vi "Humidifier CMD.vi"(8 "error in":errorcluster, 11 "cPAS in":refnum<class "cPAS.lvclass">) -> (0 "error out":errorcluster, 3 "cPAS out":refnum<class "cPAS.lvclass">)   [LabVIEW 2015, in "cPAS.lvclass"]
doc: "This VI responds to changes in the TEC Setpoint and the TEC enable for the PAS saturator. If the switch <B>RHctl</B> is set and the TEC is enabled, then the system will control the temperature setpoint based on a RH setpoint."
uses:
  cPAS.lvclass
  cPAS.lvclass/cPAS.ctl
  <vilib>/DAQmx/write.llb/DAQmx Write (Digital 1D Bool NChan 1Samp 1Line).vi
  <vilib>/DAQmx/write.llb/DAQmx Write (Analog 1D DBL NChan 1Samp).vi
  <vilib>/DAQmx/miscellaneous.llb/DAQmx Fill In Error Info.vi
  Reusable/PAS/Main/Read Data.vi
  Reusable/PAS/Data/Main/Write Current Cell.vi
  Reusable/PAS/Data/Main/Read Cell Housekeeping Data.vi
  Reusable/Humidity Control/Single Loop Humidity Control.vi
  Reusable/PAS/Data/Main/PAS Data.lvclass
  Reusable/General/Temperature/Temperature.lvlib
  Reusable/Instrument/Instrument.lvclass
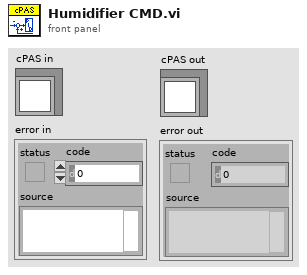
[diagram p1: front panel]
types:
  T1 = cluster{"T":sgl, "TRH":sgl, "RH":sgl, "laserRMS":sgl}
  T2 = cluster{"Array of Single[0]":sgl, "Array of Single[1]":sgl, "Array of Single[2]":sgl}
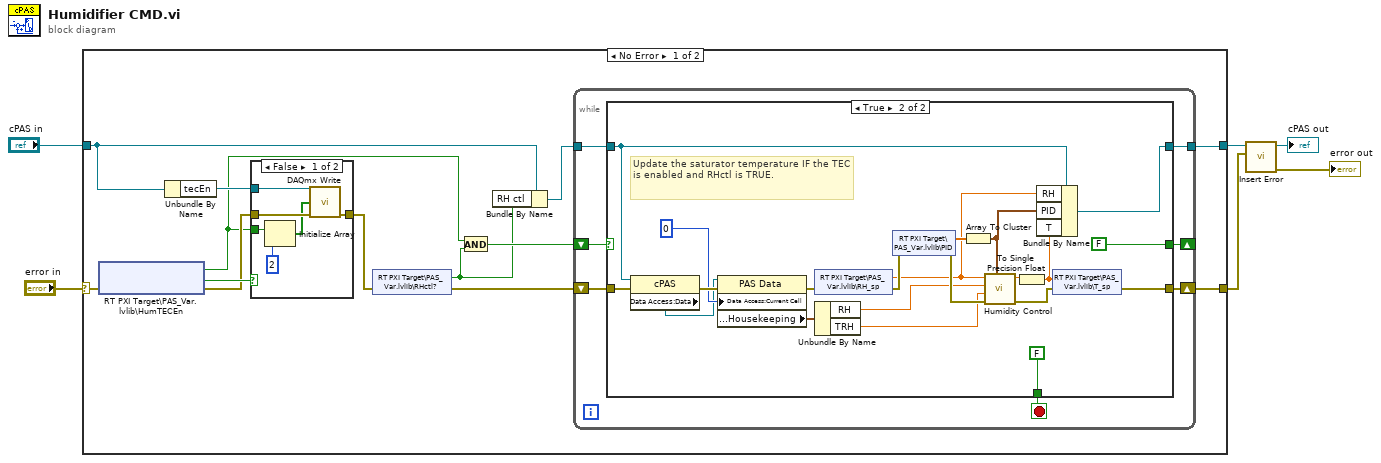
[diagram p0: block diagram]
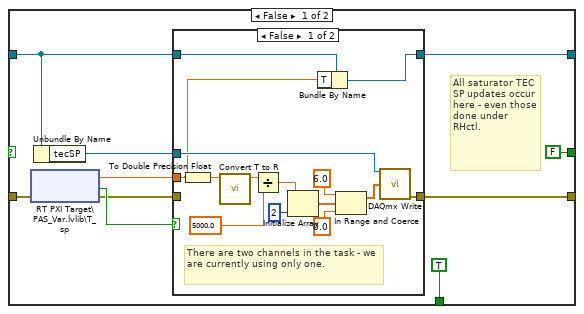
[diagram p2: hidden frame]
diagram:
  n1 = case shown="No Error" "error in" {
    selector: "error in" -> [w17 w82]
    tunnel: [w11 w82] -> w2
    tunnel: [w10 w81] -> w4
    tunnel: "cPAS in" -> [w9 w81]
    frame No Error {
      n2 = shared-variable "RT PXI Target\\PAS_Var.lvlib\\HumTECEn"(error in=w17) -> (w12:bool, error out=w16:errorcluster, w19:bool)  [unwired: 1 in]
      n3 = Unbundle By Name(w9) -> ("tecEn"=w18:refnum<k21>)
      n4 = case shown="False" w19 {
        tunnel: w18 -> [w79 _]
        tunnel: w12 -> [w76 _]
        tunnel: w16 -> [w78 w80]
        tunnel: [w77 w80] -> w13
        frame False {
          n5 = Initialize Array(w76, 2 ("dimension size")) -> (w75:bool[])
          n6 = call-poly <vilib>:"DAQmx Write.vi"("task/channels in"=w79, "data"=w75, "error in"=w78) -> ("error out"=w77:errorcluster)  [unwired: 10 in, 2 out]
        }
        frame True {
        }
      }
      n7 = shared-variable "RT PXI Target\\PAS_Var.lvlib\\RHctl?"(error in=w13) -> (w7:bool, error out=w15:errorcluster)
      n8 = And(x=w12, y=w7) -> (x .and. y?=w14:bool)
      n9 = Bundle By Name(cluster=w9, "RH ctl"=w7) -> (w8:refnum<class "cPAS.lvclass">)
      n10 = while {
        shift-right: [w24] -> w11
        shift-left: w15 -> [w23]
        tunnel: w8 -> [w22]
        shift-right: [w21] -> _
        shift-left: w14 -> [w26]
        tunnel: [w20] -> w10
        stop <- w25 stop-if-true
        n11 = case shown="True" w26 {
          tunnel: [TRUE FALSE] -> w25
          tunnel: [w32 w59] -> w24
          tunnel: w23 -> [w31 w60]
          tunnel: w22 -> [w27 w57]
          tunnel: [FALSE FALSE] -> w21
          tunnel: [w28 w54] -> w20
          frame False {
            # "All saturator TEC SP updates occur here - even those done under RHctl."
            n12 = shared-variable "RT PXI Target\\PAS_Var.lvlib\\T_sp"(error in=w31) -> (w35:sgl, error out=w33:errorcluster, w34:bool)  [unwired: 1 in]
            n13 = Unbundle By Name(w27) -> ("tecSP"=w30:refnum<k21>)
            n14 = case shown="False" w34 {
              tunnel: w30 -> [w50 _]
              tunnel: w35 -> [w38 _]
              tunnel: w33 -> [_ w52]
              tunnel: [w49 w52] -> w32
              tunnel: w27 -> [w39 w51]
              tunnel: [w37 w51] -> w28
              frame False {
                # "There are two channels in the task - we are currently using only one."
                n15 = To Double Precision Float(number=w38) -> (double precision float=w40:dbl)
                n16 = call "Convert T to R.vi"("T"=w40) -> ("R"=w46:dbl)  [unwired: 10 in]
                n17 = Divide(x=w46, y=5000.0) -> (x/y=w45:dbl)
                n18 = Initialize Array(w45, 2 ("dimension size")) -> (w44:dbl[])
                n19 = Bundle By Name(cluster=w39, "T"=w38) -> (w37:refnum<class "cPAS.lvclass">)
                n20 = In Range and Coerce(upper limit=6.0, x=w44, lower limit=0.0) -> (coerced(x)=w41:dbl[])  [unwired: 1 out]
                n21 = call-poly <vilib>:"DAQmx Write.vi"("task/channels in"=w50, "data"=w41) -> ("error out"=w49:errorcluster)  [unwired: 11 in, 2 out]
              }
              frame True {
              }
            }
          }
          frame True {
            # "Update the saturator temperature IF the TEC is enabled and RHctl is TRUE."
            n22 = property class="cPAS"(reference=w57, error in=w60) -> (error out=w67:errorcluster, "Data Access:Data"=w62:refnum<class "PAS Data.lvclass">)  [unwired: 1 out]
            n23 = property class="PAS Data"(reference=w62, error in=w67, "Data Access:Current Cell"=0 ("Current Cell")) -> (error out=w68:errorcluster, "Data Access:Housekeeping"=w64:T1)  [unwired: 1 out]
            n24 = shared-variable "RT PXI Target\\PAS_Var.lvlib\\RH_sp"(error in=w68) -> (w56:sgl, error out=w69:errorcluster)
            n25 = Unbundle By Name(w64) -> ("RH"=w65:sgl, "TRH"=w66:sgl)
            n26 = shared-variable "RT PXI Target\\PAS_Var.lvlib\\PID"(error in=w69) -> (w61:sgl[], error out=w70:errorcluster)
            n27 = Array To Cluster(array=w61) -> (cluster=w55:T2)
            n28 = call-poly "Humidity Control.vi"("PID gains"=w55, "error in"=w70, "TspIn"=w66, "RHmeas"=w65, "RHsp"=w56) -> ("error out"=w72:errorcluster, "TspOut"=w71:dbl)  [unwired: 4 in, 1 out]
            n29 = To Single Precision Float(number=w71) -> (single precision float=w53:sgl)
            n30 = Bundle By Name(cluster=w57, "RH"=w56, "PID"=w55, "T"=w53) -> (w54:refnum<class "cPAS.lvclass">)
            n31 = shared-variable "RT PXI Target\\PAS_Var.lvlib\\T_sp"(w53, error in=w72) -> (error out=w59:errorcluster)
          }
        }
      }
    }
    frame Error {
    }
  }
  n32 = call "Insert Error.vi"("err"=w2, "Instrument in"=w4) -> ("error out"=→"error out":errorcluster, "Instrument out"=→"cPAS out":refnum<class "cPAS.lvclass">)  [unwired: 7 in, 1 out]
